vi "Create Connection Handler.vi"(5 "ConnectionHandler in":refnum<class "ConnectionHandler.lvclass">, 8 "error in (no error)":errorcluster, 10 "Connection Configuration":refnum<class "Connection.lvclass">, 11 "Request":refnum<queue>) -> (0 "error out":errorcluster, 3 "ConnectionHandler":refnum<class "ConnectionHandler.lvclass">)   [LabVIEW 2013, in "MQTT Server.lvlib" / "ConnectionHandler.lvclass"]
uses:
  ConnectionHandler.lvclass
  <vilib>/LabVIEW Open Source Project/MQTT Connection/MQTT_Base/Base Class/Request -- cluster.ctl
  <vilib>/LabVIEW Open Source Project/MQTT Control Packets/Control Packets/ControlPacket/ControlPacket.lvclass
  <vilib>/LabVIEW Open Source Project/MQTT Connection/MQTT_Base/Base Class/Response -- cluster.ctl
  <vilib>/LabVIEW Open Source Project/MQTT Connection/MQTT_Connection/Connection/Connection.lvclass
  ConnectionHandler.lvclass/ConnectionHandler.ctl
  <vilib>/LabVIEW Open Source Project/MQTT Connection/MQTT_Base/Base Class/MQTT_Base.lvclass
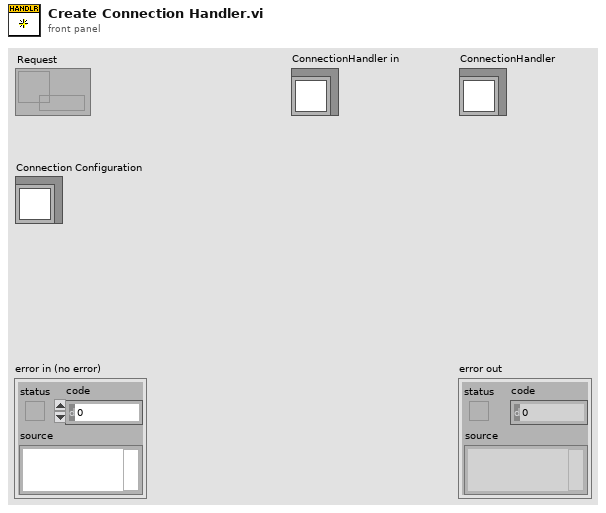
[diagram p1: front panel]
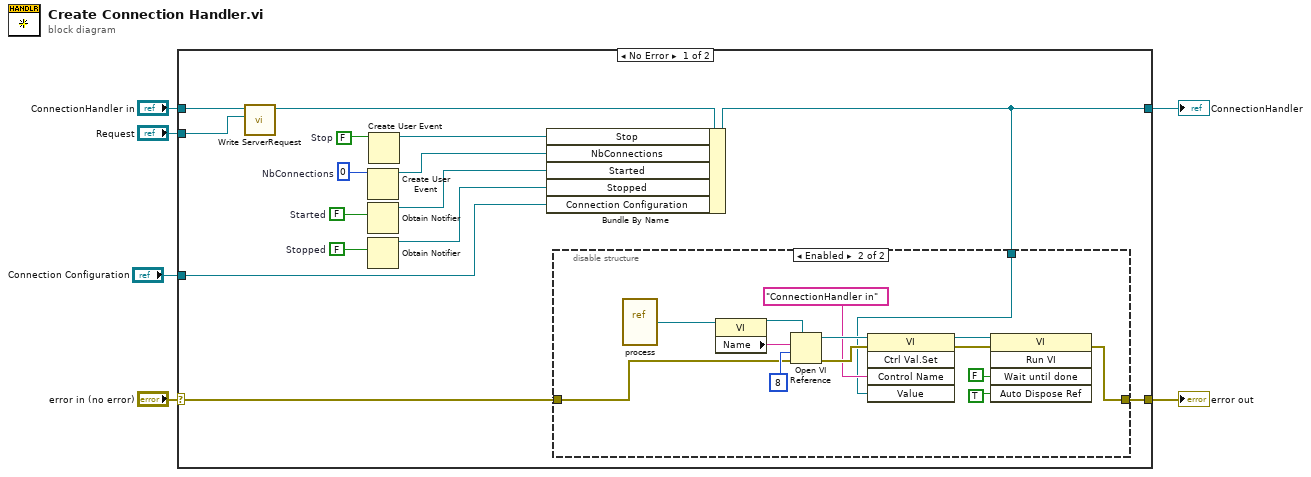
[diagram p0: block diagram]
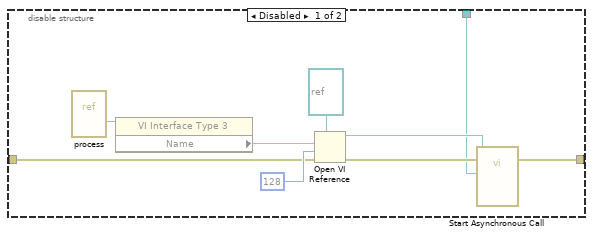
[diagram p2: hidden frame]
diagram:
  n1 = case shown="No Error" "error in (no error)" {
    selector: "error in (no error)" -> [w13 w46]
    tunnel: [w12 w46] -> w5
    tunnel: [w16 w45] -> w3
    tunnel: "ConnectionHandler in" -> [w20 w45]
    tunnel: "Request" -> [w21 _]
    tunnel: "Connection Configuration" -> [w7 _]
    frame No Error {
      w11 = u32 0  # NbConnections
      w14 = FALSE  # Stopped
      w15 = FALSE  # Started
      w19 = FALSE  # Stop
      n2 = call "Write ServerRequest.vi"("ServerRequest"=w21, "TCPConnectionHandler in"=w20) -> ("TCPConnectionHandler out"=w17:refnum<class "ConnectionHandler.lvclass">)  [unwired: 9 in]
      n3 = Create User Event(user event datatype=w11) -> (user event=w10:refnum<user-event>)  [unwired: 1 in, 1 out]
      n4 = Obtain Notifier(notification data type=w15) -> (notifier out=w9:refnum<notifier>)  [unwired: 3 in, 2 out]
      n5 = Obtain Notifier(notification data type=w14) -> (notifier out=w8:refnum<notifier>)  [unwired: 3 in, 2 out]
      n6 = Create User Event(user event datatype=w19) -> (user event=w18:refnum<user-event>)  [unwired: 1 in, 1 out]
      n7 = Bundle By Name(cluster=w17, "Stop"=w18, "NbConnections"=w10, "Started"=w9, "Stopped"=w8, "Connection Configuration"=w7) -> (w16:refnum<class "ConnectionHandler.lvclass">)
      n8 = disable-structure shown="Enabled" {
        disable-tunnel: w16 -> [w25 w31]
        disable-tunnel: w13 -> [w24 w32]
        disable-tunnel: [w23 w33] -> w12
        frame Disabled {
          n9 = vi-ref "process.vi"() -> (w30:refnum<vi>)
          n10 = property class="VI Interface Type 3"(reference=w30) -> ("Name"=w29:string)  [unwired: 1 in, 2 out]
          n11 = Open VI Reference(type specifier VI Refnum (for type only)=refnum<vi> refnum ("reference out"), vi path=w29, options=128, error in (no error)=w24) -> (vi reference=w28:refnum<vi>, error out=w27:errorcluster)  [unwired: 2 in]
          n12 = call-by-ref "Start Asynchronous Call"(reference=w28, error in=w27, "ConnectionHandler in"=w25) -> (error out=w23:errorcluster)  [unwired: 9 in, 3 out]
        }
        frame Enabled {
          n13 = vi-ref "process.vi"() -> (w34:refnum<vi>)
          n14 = property class="VI"(reference=w34) -> (reference out=w43:refnum<vi>, "Name"=w44:string)  [unwired: 1 in, 1 out]
          n15 = Open VI Reference(type specifier VI Refnum (for type only)=w43, vi path=w44, options=8, error in (no error)=w32) -> (vi reference=w36:refnum<vi>, error out=w37:errorcluster)  [unwired: 2 in]
          n16 = invoke class="VI" method="Ctrl Val.Set"(reference=w36, error in=w37, "Control Name"="ConnectionHandler in", "Value"=w31) -> (reference out=w40:refnum<vi>, error out=w41:errorcluster)  [unwired: 1 in, 3 out]
          n17 = invoke class="VI" method="Run VI"(reference=w40, error in=w41, "Wait until done"=FALSE ("Wait Until Done"), "Auto Dispose Ref"=TRUE ("Auto Dispose Reference")) -> (error out=w33:errorcluster)  [unwired: 1 in, 4 out]
        }
      }
    }
    frame Error {
    }
  }
  "error out" <- w5
  "ConnectionHandler" <- w3
